vi "Configure Modulation(FSK).vi"(0 "VISA resource name":refnum<visa-resource-name>, 1 "Enable FSK Modulation (F: Disable)":bool, 5 "Channel (1: Channel 1)":i32(ring)=1 items=["Channel 1"=1, "Channel 2"=2], 7 "FSK Source (0: Internal)":i32(ring) items=["Internal", "External"], 9 "Modulating Polarity (0: Positive)":i32(ring) items=["Positive", "Negative"], 11 "error in (no error)":errorcluster, 12 "Hop Frequency (100 Hz)":dbl=100.0, 13 "FSK Rate (100 Hz)":dbl=100.0) -> (4 "VISA resource name out":refnum<visa-resource-name>, 15 "error out":errorcluster)   [LabVIEW 2012, in "RIGOL DG4000 Series.lvlib"]
doc: "Configures FSK (Frequency Shifting Keying) modulation."
uses:
  <instrlib>/RIGOL DG4000 Series/RIGOL DG4000 Series.lvlib
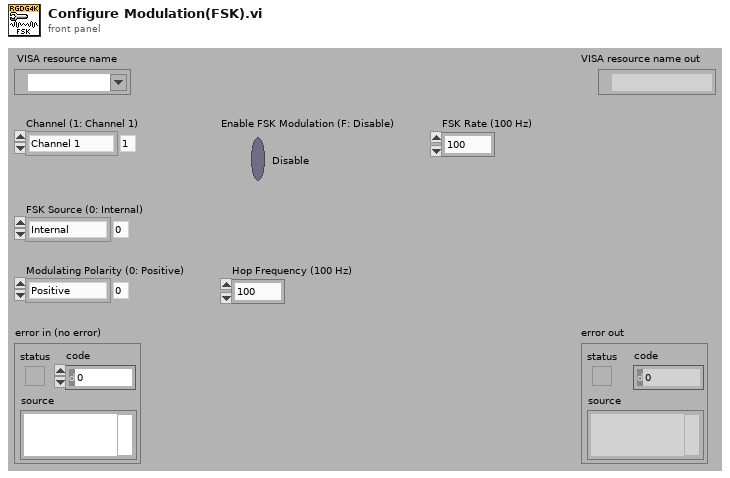
[diagram p1: front panel]
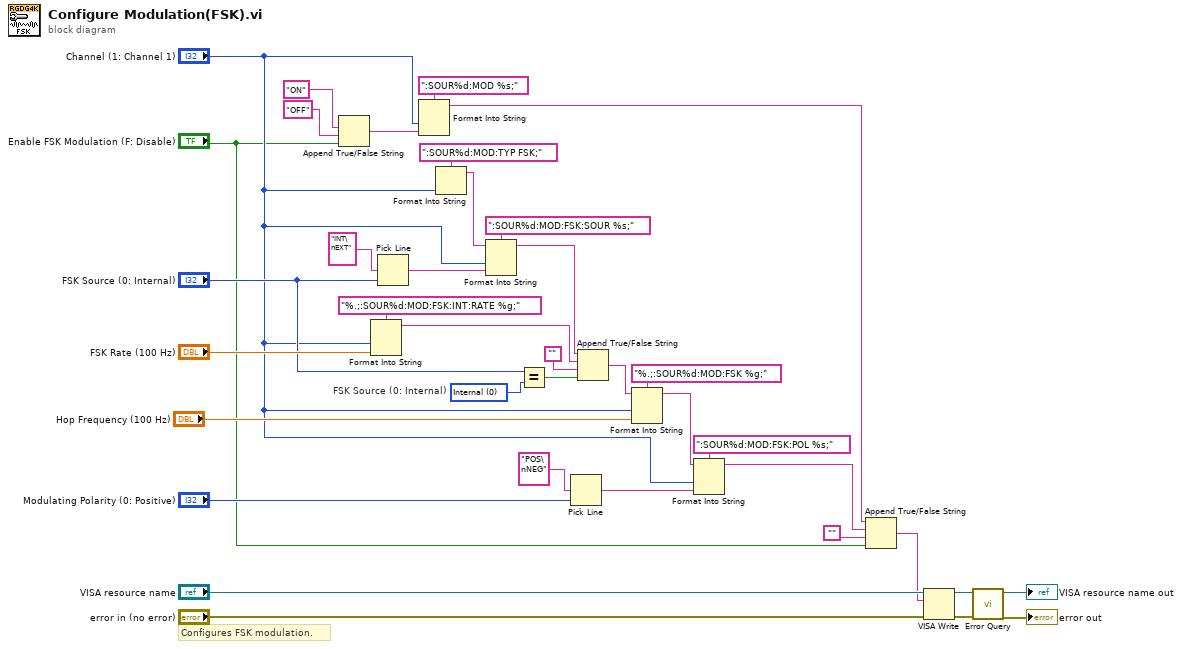
[diagram p0: block diagram]
diagram:
  w10 = 0 items=["Internal", "External"]  # FSK Source (0: Internal)
  # "Configures FSK modulation."
  n1 = Append True/False String(1:"Enable FSK Modulation (F: Disable)", 2:"OFF", 3:"ON") -> (0:w34:string)  [unwired: 1 out]
  n2 = Format Into String(format string="%.;:SOUR%d:MOD:FSK:INT:RATE %g;", "Channel (1: Channel 1)", "FSK Rate (100 Hz)") -> (resulting string=w13:string)  [unwired: 2 in, 1 out]
  n3 = Pick Line(multi-line string="INT\nEXT", line index="FSK Source (0: Internal)") -> (output string=w29:string)  [unwired: 1 out]
  n4 = Format Into String(format string=":SOUR%d:MOD %s;", "Channel (1: Channel 1)", w34) -> (resulting string=w4:string)  [unwired: 2 in, 1 out]
  n5 = Format Into String(format string=":SOUR%d:MOD:TYP FSK;", "Channel (1: Channel 1)") -> (resulting string=w31:string)  [unwired: 2 in, 1 out]
  n6 = Format Into String(format string=":SOUR%d:MOD:FSK:SOUR %s;", initial string=w31, "Channel (1: Channel 1)", w29) -> (resulting string=w15:string)  [unwired: 1 in, 1 out]
  n7 = Equal?(x="FSK Source (0: Internal)", y=w10) -> (x = y?=w12:bool)
  n8 = Pick Line(multi-line string="POS\nNEG", line index="Modulating Polarity (0: Positive)") -> (output string=w22:string)  [unwired: 1 out]
  n9 = Append True/False String(1:w12, 2:"", 3:w13, 4:w15) -> (0:w7:string)
  n10 = Format Into String(format string="%.;:SOUR%d:MOD:FSK %g;", initial string=w7, "Channel (1: Channel 1)", "Hop Frequency (100 Hz)") -> (resulting string=w6:string)  [unwired: 1 in, 1 out]
  n11 = Format Into String(format string=":SOUR%d:MOD:FSK:POL %s;", initial string=w6, "Channel (1: Channel 1)", w22) -> (resulting string=w3:string)  [unwired: 1 in, 1 out]
  n12 = Append True/False String(1:"Enable FSK Modulation (F: Disable)", 2:"", 3:w3, 4:w4) -> (0:w1:string)
  n13 = VISA Write(VISA resource name="VISA resource name", write buffer=w1, error in (no error)="error in (no error)") -> (VISA resource name out=w19:refnum<visa-resource-name>, error out=w18:errorcluster)  [unwired: 1 out]
  n14 = call <instrlib>:"Error Query.vi"("error in (no error)"=w18, "VISA resource name"=w19) -> ("error out"=→"error out":errorcluster, "VISA resource name out"=→"VISA resource name out":refnum<visa-resource-name>)  [unwired: 8 out]
